vi "Programming Example Terahertz StepScan and FastScan.vi"() -> ()   [LabVIEW 2013]
uses:
  SubVIs/DeCoF SubVI Library/subVIs/DeCoF connection.ctl
  SubVIs/Commands.ctl
  SubVIs/Measurement.ctl
  SubVIs/Variables.ctl
  SubVIs/Store Data Actions.ctl
panel:
  in  "Set Bias to Zero":bool
  in  "Set Bias to Default":bool
  in  "IP Address of DLC smart":string="192.168.54.80"
  in  "Send All Values to DLC smart":bool
  out "Points Read":i32
  out "Fast-Scan-IsScanning":bool
  in  "FastScan":bool
  in  "Tx Amplitude":dbl caption="Tx Bias Amplitude (V)" step=0.1 format="%#.6g"
  in  "Tx Offset":dbl caption="Tx Bias Offset (V)" step=0.1 format="%#.6g"
  out "DLC smart Info":string
  in  "Int-Time(ms)":dbl=3.2768 caption="Integration Time (ms)" format="%#.6g"
  out "DLC smart Ok?":bool
  in  "Continuously":bool
  in  "Scan Selection":enum32{"No Selection", "Scan Up", "Scan Down"}(radio)
  in  "Quit App":bool
  in  "Max":dbl=650.0 caption="Max (GHz)"
  out "act.Step":dbl
  out "Graph Scan":T1(graph)
  in  "Step":dbl=0.002 caption="Step (GHz)" min=0.0 step=1e-05 format="%#_6f"
  in  "Min":dbl=600.0 caption="Min (GHz)"
  in  "Save Graph":bool
  in  "Clear Graph":bool
  out "Graph Samp":dbl[](graph)
  out "THz Cur":dbl caption="THz Current (nA)"
  in  "Gain Transimp. Amp.":dbl(ring)=1000000.0 caption="Transimp. Amp. Gain" items=["10^3 V/A"=1000.0, "10^4 V/A"=10000.0, "3.3 10^4 V/A  (1)"=33000.0, "10^5 V/A  (2)"=100000.0, "3.3 10^5 V/A  (3)"=330000.0, "10^6 V/A  (4)"=1000000.0, "3.3 10^6 V/A  (5)"=3300000.0, "10^7 V/A  (6)"=10000000.0]
  out "Connected?":bool
  in  "Sampling":bool
  in  "Freq.":dbl=600.0 caption="Frequency (GHz)" format="%#.6g"
  out "Connection ID":T2
  in  "Connect to DLC smart":bool
  in  "Laser Emission OnOff":bool
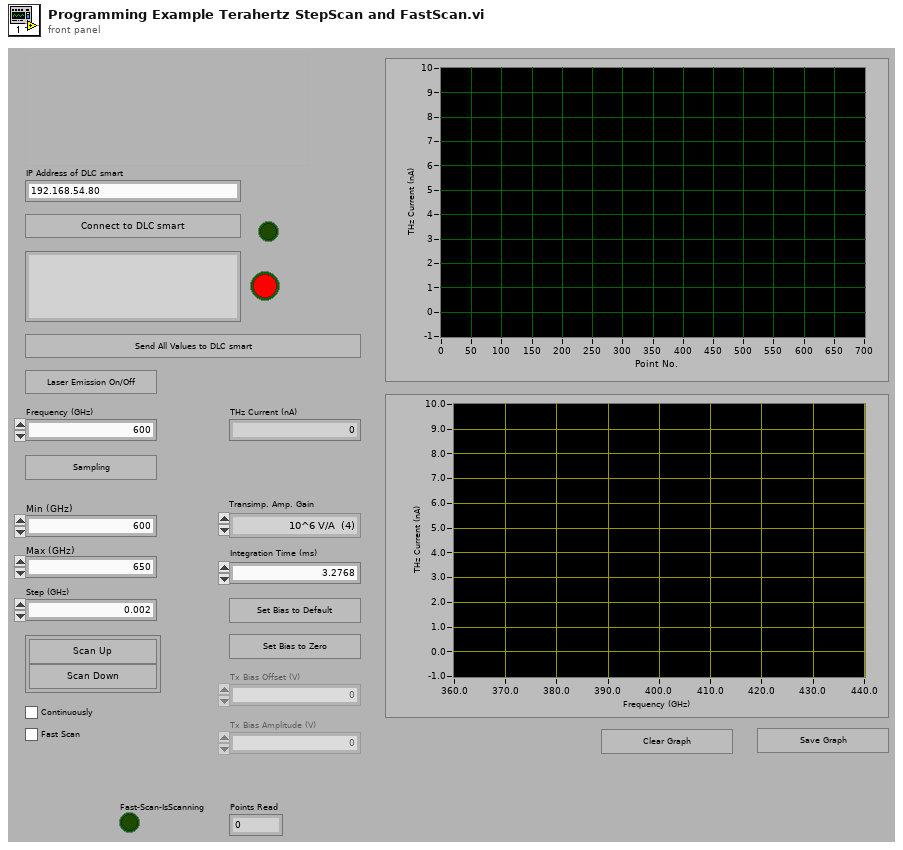
[diagram p1: front panel]
types:
  T1 = cluster{"array w/ subset deleted":dbl[], "array w/ subset deleted":dbl[]}
  T2 = typedef "DeCoF connection.ctl" = cluster{"TCP/IP":bool, "VISA":refnum<visa-resource-name>, "TCP/IP ID":refnum<k5>}
  T3 = typedef "Measurement.ctl" = enum16{"Init System", "Start Sampling", "Start Scan", "FastScan - Start", "FastScan - Get Data", "FastScan - Plot", "FastScan - End of Loop", "Precise - Set Frequency", "Precise - Reset Lock-In", "Precise - Wait", "Precise - Read Lock-In", "Precise - Store Data", "Precise - Plot", "Precise - End of Loop", "Stop Loop"}
  T4 = typedef "Commands.ctl" = enum16{"Init System", "Connect to DLC smart", "Verify DLC smart", "Laser Emission", "Send All Values to DLC smart", "Set Frequency", "Set FrequencyMin", "Set FrequencyMax", "Set FrequencyStep", "Set ScanModeFast", "Integration Time", "Set Bias to Default", "Set Bias to Zero", "Tx Bias Voltage", "Clear Graph", "Save Graph", "Clean Up"}
  T5 = typedef "Store Data Actions.ctl" = enum16{"Init", "Set", "Add", "Add Array", "Read", "Row+N"}
  T6 = typedef "Variables.ctl" = i32
  T7 = enum32{"invalid app kind", "Development System", "Run Time System", "Student Edition", "Embedded LabVIEW", "Evaluation", "Custom"}
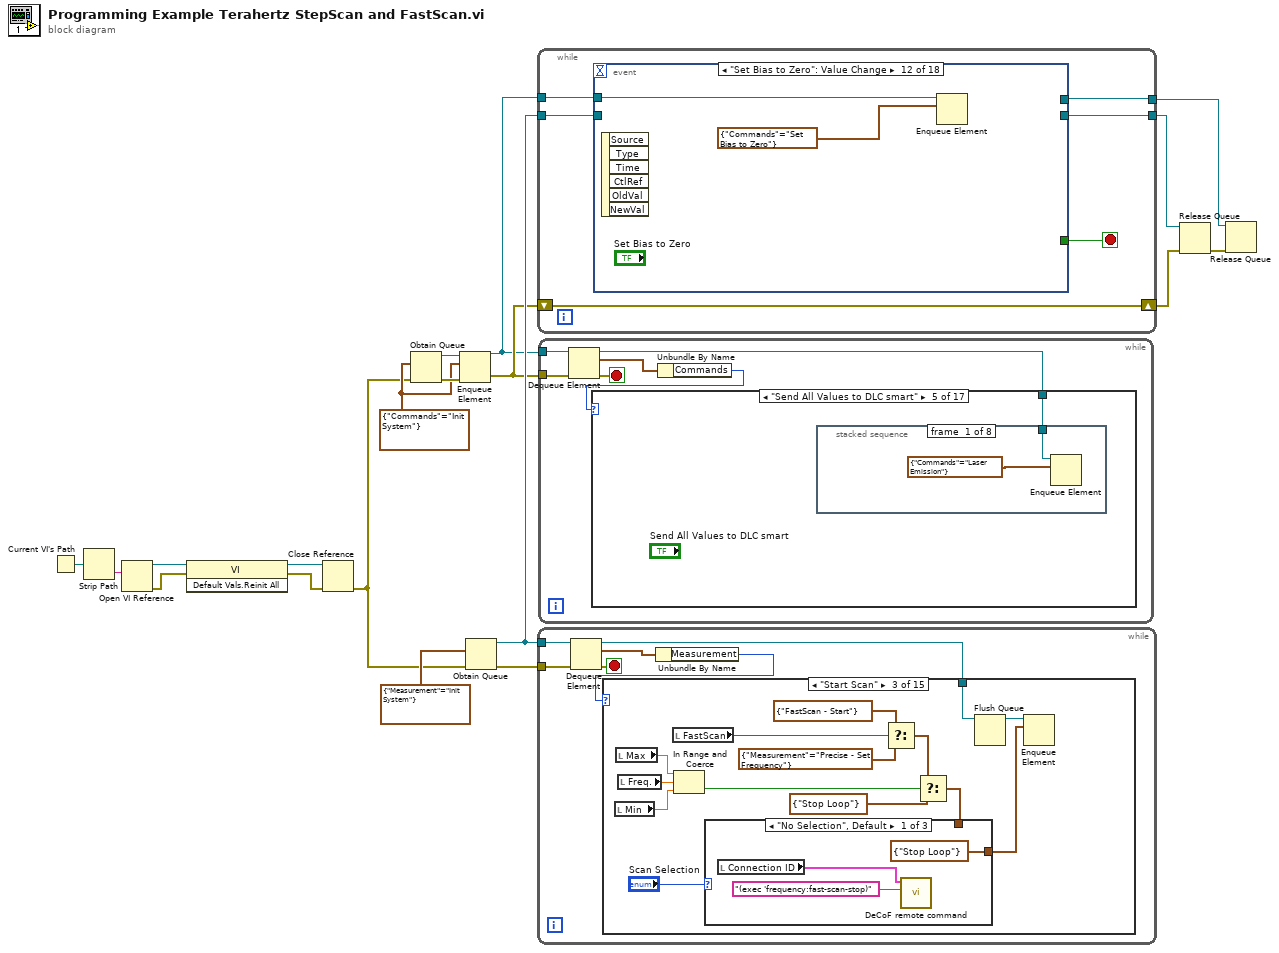
[diagram p0: block diagram]
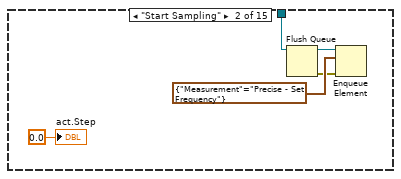
[diagram p3: hidden frame]
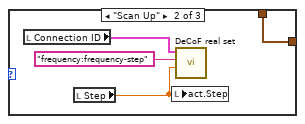
[diagram p4: hidden frame]
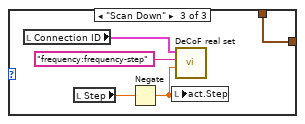
[diagram p5: hidden frame]
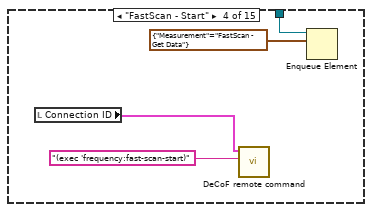
[diagram p6: hidden frame]
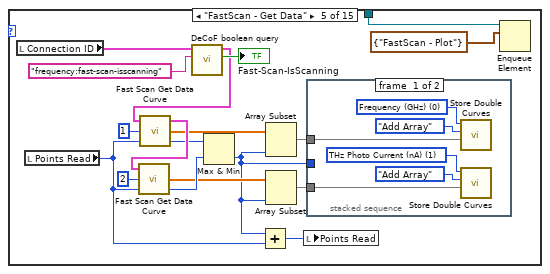
[diagram p7: hidden frame]
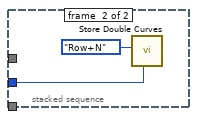
[diagram p8: hidden frame]
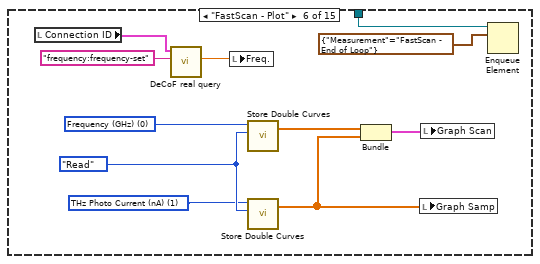
[diagram p9: hidden frame]
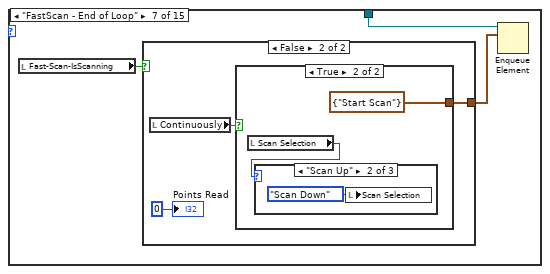
[diagram p10: hidden frame]
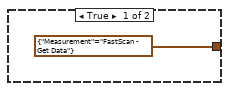
[diagram p11: hidden frame]
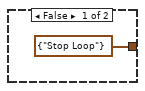
[diagram p12: hidden frame]
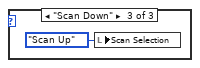
[diagram p14: hidden frame]
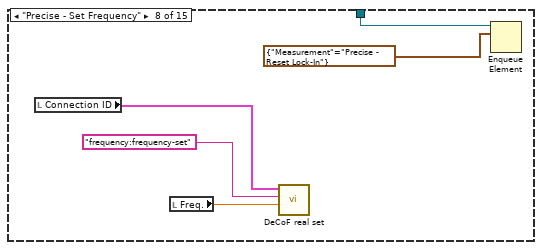
[diagram p15: hidden frame]
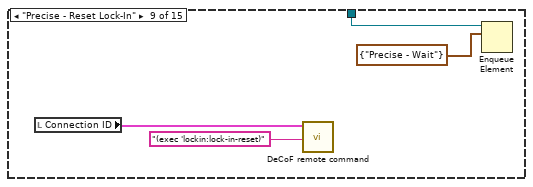
[diagram p16: hidden frame]
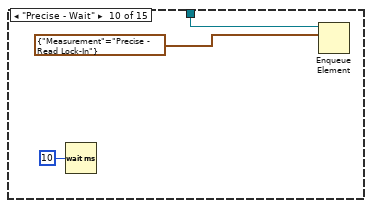
[diagram p17: hidden frame]
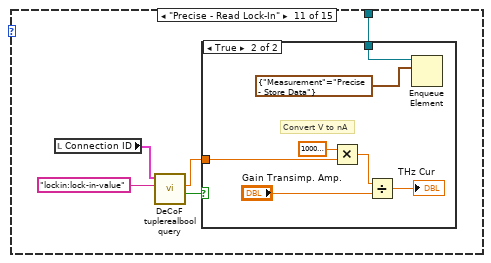
[diagram p18: hidden frame]
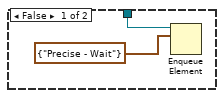
[diagram p19: hidden frame]
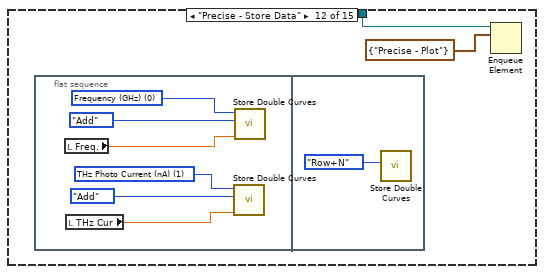
[diagram p20: hidden frame]
diagram:
  w16 = cluster{"Commands":T4} {"Commands"=enum."Init System"}
  n1 = Current VI's Path() -> (path=w10:path)
  n2 = Strip Path(path=w10) -> (name=w11:string)  [unwired: 1 out]
  n3 = Open VI Reference(vi path=w11) -> (vi reference=w9:refnum<vi>, error out=w13:errorcluster)  [unwired: 5 in]
  n4 = invoke class="VI" method="Default Vals.Reinit All"(reference=w9, error in=w13) -> (reference out=w12:refnum<vi>, error out=w14:errorcluster)  [unwired: 1 in, 1 out]
  n5 = Close Reference(reference=w12, error in (no error)=w14) -> (error out=w8:errorcluster)
  n6 = Obtain Queue(element data type=w16, error in (no error)=w8) -> (queue out=w19:refnum<queue>, error out=w18:errorcluster)  [unwired: 3 in, 1 out]
  n7 = Enqueue Element(queue=w19, element=w16, error in (no error)=w18) -> (queue out=w1:refnum<queue>, error out=w6:errorcluster)  [unwired: 1 in, 1 out]
  n8 = Obtain Queue(element data type=cluster{"Measurement":T3} {"Measurement"=enum."Init System"}, error in (no error)=w8) -> (queue out=w7:refnum<queue>, error out=w17:errorcluster)  [unwired: 3 in, 1 out]
  n9 = while {
    tunnel: w7 -> [w25]
    shift-right: [w21] -> w2
    shift-left: w6 -> [w21]
    tunnel: [w23] -> w4
    tunnel: [w22] -> w3
    tunnel: w1 -> [w20]
    stop <- w24 stop-if-true
    n10 = event shown="[11] \"Set Bias to Zero\": Value Change" {
      selector: _ -> [_ _ _ _ _ _ _ _ _ _ _ _ _ _ _ _ _ _]
      dyn-events: _ -> [_ _ _ _ _ _ _ _ _ _ _ _ _ _ _ _ _ _]
      timeout: _ -> [_ _ _ _ _ _ _ _ _ _ _ _ _ _ _ _ _ _]
      tunnel: w25 -> [_ _ _ _ _ _ _ _ _ _ _ _ _ w57 w60 _ _ w67]
      tunnel: [_ _ _ _ _ _ _ _ _ _ _ _ _ _ _ _ _ "Quit App"] -> w24
      tunnel: [_ _ _ _ _ _ _ _ _ _ _ _ _ _ _ _ _ w67] -> w23
      tunnel: [_ _ _ _ _ _ _ _ _ _ _ _ _ _ _ _ _ w66] -> w22
      tunnel: w20 -> [w26 w28 w30 w32 w34 w36 w38 w40 w42 w44 w46 w48 w50 _ _ w61 w63 w66]
      event "Connect to DLC smart": Value Change {
        n11 = event-data() -> ()  [unwired: 1 in, 5 out]
        n12 = Enqueue Element(queue=w26, element=cluster{"Commands":T4} {"Commands"=enum."Connect to DLC smart"}) -> ()  [unwired: 2 in, 3 out]
      }
      event "Save Graph": Value Change {
        n13 = event-data() -> ()  [unwired: 1 in, 5 out]
        n14 = Enqueue Element(queue=w28, element=cluster{"Commands":T4} {"Commands"=enum."Save Graph"}) -> ()  [unwired: 2 in, 3 out]
      }
      event "Laser Emission OnOff": Value Change {
        n15 = event-data() -> ()  [unwired: 1 in, 6 out]
        n16 = Enqueue Element(queue=w30, element=cluster{"Commands":T4} {"Commands"=enum."Laser Emission"}) -> ()  [unwired: 2 in, 3 out]
      }
      event "Send All Values to DLC smart": Value Change {
        n17 = event-data() -> ()  [unwired: 1 in, 6 out]
        n18 = Enqueue Element(queue=w32, element=cluster{"Commands":T4} {"Commands"=enum."Send All Values to DLC smart"}) -> ()  [unwired: 2 in, 3 out]
      }
      event "Freq.": Value Change {
        n19 = event-data() -> ()  [unwired: 1 in, 6 out]
        n20 = Enqueue Element(queue=w34, element=cluster{"Commands":T4} {"Commands"=enum."Set Frequency"}) -> ()  [unwired: 2 in, 3 out]
      }
      event "Min": Value Change {
        n21 = event-data() -> ()  [unwired: 1 in, 6 out]
        n22 = Enqueue Element(queue=w36, element=cluster{"Commands":T4} {"Commands"=enum."Set FrequencyMin"}) -> ()  [unwired: 2 in, 3 out]
      }
      event "Max": Value Change {
        n23 = event-data() -> ()  [unwired: 1 in, 6 out]
        n24 = Enqueue Element(queue=w38, element=cluster{"Commands":T4} {"Commands"=enum."Set FrequencyMax"}) -> ()  [unwired: 2 in, 3 out]
      }
      event "Step": Value Change {
        n25 = event-data() -> ()  [unwired: 1 in, 6 out]
        n26 = Enqueue Element(queue=w40, element=cluster{"Commands":T4} {"Commands"=enum."Set FrequencyStep"}) -> ()  [unwired: 2 in, 3 out]
      }
      event "FastScan": Value Change {
        n27 = event-data() -> ()  [unwired: 1 in, 6 out]
        n28 = Enqueue Element(queue=w42, element=cluster{"Commands":T4} {"Commands"=enum."Set ScanModeFast"}) -> ()  [unwired: 2 in, 3 out]
      }
      event "Int-Time(ms)": Value Change {
        n29 = event-data() -> ()  [unwired: 1 in, 6 out]
        n30 = Enqueue Element(queue=w44, element=cluster{"Commands":T4} {"Commands"=enum."Integration Time"}) -> ()  [unwired: 2 in, 3 out]
      }
      event "Set Bias to Default": Value Change {
        n31 = event-data() -> ()  [unwired: 1 in, 6 out]
        n32 = Enqueue Element(queue=w46, element=cluster{"Commands":T4} {"Commands"=enum."Set Bias to Default"}) -> ()  [unwired: 2 in, 3 out]
      }
      event "Set Bias to Zero": Value Change {
        n33 = event-data() -> ()  [unwired: 1 in, 6 out]
        n34 = Enqueue Element(queue=w48, element=cluster{"Commands":T4} {"Commands"=enum."Set Bias to Zero"}) -> ()  [unwired: 2 in, 3 out]
      }
      event "Tx Offset", "Tx Amplitude": Value Change {
        n35 = event-data() -> ()  [unwired: 1 in, 6 out]
        n36 = Enqueue Element(queue=w50, element=cluster{"Commands":T4} {"Commands"=enum."Tx Bias Voltage"}) -> ()  [unwired: 2 in, 3 out]
      }
      event "Sampling": Value Change {
        n37 = event-data() -> ("NewVal"=w56:bool)  [unwired: 1 in, 5 out]
        n38 = local write "Scan Selection"(enum32{"No Selection", "Scan Up", "Scan Down"}."No Selection" ("Scan Selection")) -> ()
        n39 = Select(t=cluster{"Measurement":T3} {"Measurement"=enum."Start Sampling"}, s=w56, f=cluster{"Measurement":T3} {"Measurement"=enum."Stop Loop"} ("element")) -> (s? t:f=w54:cluster{"Measurement":T3})
        n40 = Enqueue Element(queue=w57, element=w54) -> ()  [unwired: 2 in, 3 out]
      }
      event "Scan Selection": Value Change {
        n41 = event-data() -> ()  [unwired: 1 in, 6 out]
        n42 = local write "Sampling"(FALSE ("Start Scan UI")) -> ()
        n43 = Enqueue Element(queue=w60, element=cluster{"Measurement":T3} {"Measurement"=enum."Start Scan"}) -> ()  [unwired: 2 in, 3 out]
      }
      event "Clear Graph": Value Change {
        n44 = event-data() -> ()  [unwired: 1 in, 5 out]
        n45 = Enqueue Element(queue=w61, element=cluster{"Commands":T4} {"Commands"=enum."Clear Graph"}) -> ()  [unwired: 2 in, 3 out]
      }
      event Panel Close? {
        n46 = event-data() -> ()  [unwired: 1 in, 3 out]
        n47 = Enqueue Element(queue=w63, element=cluster{"Commands":T4} {"Commands"=enum."Clean Up"}) -> ()  [unwired: 2 in, 3 out]
        n48 = event-data("Discard?"=TRUE ("stop")) -> ()  [unwired: 1 in, 1 out]
      }
      event "Quit App": Value Change {
        n49 = event-data() -> ()  [unwired: 1 in, 5 out]
      }
    }
  }
  n50 = while {
    tunnel: w7 -> [w74]
    tunnel: w17 -> [w73]
    stop <- w72 stop-if-true
    n51 = Dequeue Element(queue=w74, error in (no error)=w73) -> (queue out=w70:refnum<queue>, element=w69:cluster{"Measurement":T3}, error out=w72:errorcluster)  [unwired: 1 in, 1 out]
    n52 = Unbundle By Name(w69) -> ("Measurement"=w71:T3)
    n53 = case shown="\"Start Scan\"" w71 {
      tunnel: w70 -> [_ w78 w93 w109 w127 w146 w149 w162 w165 w169 w175 w186 w201 w211 w224]
      frame "Init System" {
      }
      frame "Start Sampling" {
        n54 = Flush Queue(queue=w78) -> (queue out=w77:refnum<queue>, error out=w76:errorcluster)  [unwired: 1 in, 1 out]
        n55 = Enqueue Element(queue=w77, element=cluster{"Measurement":T3} {"Measurement"=enum."Precise - Set Frequency"}, error in (no error)=w76) -> ()  [unwired: 1 in, 3 out]
        "act.Step" <- 0.0 ("act.Step")
      }
      frame "Start Scan" {
        n56 = local read "Min"() -> (w89:dbl)
        n57 = local read "Max"() -> (w90:dbl)
        n58 = local read "Freq."() -> (w91:dbl)
        n59 = local read "FastScan"() -> (w83:bool)
        n60 = In Range and Coerce(upper limit=w90, x=w91, lower limit=w89) -> (In Range?=w87:bool)  [unwired: 1 out]
        n61 = Select(t=cluster{"Measurement":T3} {"Measurement"=enum."FastScan - Start"}, s=w83, f=cluster{"Measurement":T3} {"Measurement"=enum."Precise - Set Frequency"} ("element")) -> (s? t:f=w86:cluster{"Measurement":T3})
        n62 = Select(t=w86, s=w87, f=cluster{"Measurement":T3} {"Measurement"=enum."Stop Loop"} ("element")) -> (s? t:f=w82:cluster{"Measurement":T3})
        n63 = case shown="\"No Selection\", Default" "Scan Selection" {
          tunnel: w82 -> [_ w100 w104]
          tunnel: [cluster{"Measurement":T3} {"Measurement"=enum."Stop Loop"} ("element") w100 w104] -> w81
          frame "No Selection", Default {
            n64 = local read "Connection ID"() -> (w94:T2)
            n65 = call "DeCoF remote command.vi"("command"="(exec 'frequency:fast-scan-stop)" ("param-name"), "Conncection ID in"=w94) -> ()  [unwired: 3 in, 5 out]
          }
          frame "Scan Up" {
            n66 = local read "Connection ID"() -> (w98:T2)
            n67 = local read "Step"() -> (w97:dbl)
            n68 = local write "act.Step"(w97) -> ()
            n69 = call "DeCoF real set.vi"("value"=w97, "param-name"="frequency:frequency-step", "Conncection ID in"=w98) -> ()  [unwired: 3 in, 2 out]
          }
          frame "Scan Down" {
            n70 = local read "Connection ID"() -> (w102:T2)
            n71 = local read "Step"() -> (w105:dbl)
            n72 = Negate(x=w105) -> (-x=w101:dbl)
            n73 = local write "act.Step"(w101) -> ()
            n74 = call "DeCoF real set.vi"("value"=w101, "param-name"="frequency:frequency-step", "Conncection ID in"=w102) -> ()  [unwired: 3 in, 2 out]
          }
        }
        n75 = Flush Queue(queue=w93) -> (queue out=w92:refnum<queue>)  [unwired: 1 in, 2 out]
        n76 = Enqueue Element(queue=w92, element=w81) -> ()  [unwired: 2 in, 3 out]
      }
      frame "FastScan - Start" {
        n77 = local read "Connection ID"() -> (w106:T2)
        n78 = call "DeCoF remote command.vi"("command"="(exec 'frequency:fast-scan-start)" ("param-name"), "Conncection ID in"=w106) -> ()  [unwired: 3 in, 5 out]
        n79 = Enqueue Element(queue=w109, element=cluster{"Measurement":T3} {"Measurement"=enum."FastScan - Get Data"}) -> ()  [unwired: 2 in, 3 out]
      }
      frame "FastScan - Get Data" {
        n80 = local read "Connection ID"() -> (w126:T2)
        n81 = local read "Points Read"() -> (w112:i32)
        n82 = call "DeCoF boolean query.vi"("param-name"="frequency:fast-scan-isscanning", "Conncection ID in"=w126) -> ("value"=→"Fast-Scan-IsScanning":bool, "Conncection ID out"=w122:T2)  [unwired: 3 in, 1 out]
        n83 = call "Fast Scan Get Data Curve.vi"("Start Index"=w112, "Curve Number"=1, "Conncection ID in"=w122) -> ("Size of Double Array"=w118:i32, "Double Array"=w116:dbl[], "Conncection ID out"=w120:T2)
        n84 = call "Fast Scan Get Data Curve.vi"("Start Index"=w112, "Curve Number"=2, "Conncection ID in"=w120) -> ("Size of Double Array"=w117:i32, "Double Array"=w115:dbl[])  [unwired: 1 out]
        n85 = Max & Min(x=w118, y=w117) -> (min(x,y)=w110:i32)  [unwired: 1 out]
        n86 = Add(x=w110, y=w112) -> (x+y=w111:i32)
        n87 = Array Subset(array=w116, length=w110) -> (w114:dbl[])  [unwired: 1 in]
        n88 = Array Subset(array=w115, length=w110) -> (w113:dbl[])  [unwired: 1 in]
        n89 = local write "Points Read"(w111) -> ()
        n90 = stacked-sequence {
          tunnel: w114 -> [w133 _]
          tunnel: w113 -> [w128 _]
          tunnel: w110 -> [_ w134]
          frame #0 {
            w130 = T6 1 items=["Frequency (GHz)", "THz Photo Current (nA)"] ("Curve Index")
            w131 = T6 0 items=["Frequency (GHz)", "THz Photo Current (nA)"] ("Curve Index")
            n91 = call "Store Double Curves.vi"("Array in"=w133, "Action"=Store_Data_Actions."Add Array", "Curve Index"=w131) -> ()  [unwired: 3 in, 2 out]
            n92 = call "Store Double Curves.vi"("Array in"=w128, "Action"=Store_Data_Actions."Add Array", "Curve Index"=w130) -> ()  [unwired: 3 in, 2 out]
          }
          frame #1 {
            n93 = call "Store Double Curves.vi"("N"=w134, "Action"=Store_Data_Actions."Row+N") -> ()  [unwired: 4 in, 2 out]
          }
        }
        n94 = Enqueue Element(queue=w127, element=cluster{"Measurement":T3} {"Measurement"=enum."FastScan - Plot"}) -> ()  [unwired: 2 in, 3 out]
      }
      frame "FastScan - Plot" {
        w142 = T6 0 items=["Frequency (GHz)", "THz Photo Current (nA)"] ("Curve Index")
        w143 = T6 1 items=["Frequency (GHz)", "THz Photo Current (nA)"] ("Curve Index")
        w144 = Store_Data_Actions."Read" ("Action")
        n95 = local read "Connection ID"() -> (w138:T2)
        n96 = call "DeCoF real query.vi"("param-name"="frequency:frequency-set", "Conncection ID in"=w138) -> ("value"=w136:dbl)  [unwired: 3 in, 2 out]
        n97 = local write "Freq."(w136) -> ()
        n98 = call "Store Double Curves.vi"("Action"=w144, "Curve Index"=w142) -> ("Array out"=w141:dbl[])  [unwired: 4 in, 1 out]
        n99 = call "Store Double Curves.vi"("Action"=w144, "Curve Index"=w143) -> ("Array out"=w139:dbl[])  [unwired: 4 in, 1 out]
        n100 = Bundle("Array out"=w141, "Array out"=w139) -> (w140:cluster{"Array out":dbl[], "Array out":dbl[]})  [unwired: 1 in]
        n101 = local write "Graph Samp"(w139) -> ()
        n102 = local write "Graph Scan"(w140) -> ()
        n103 = Enqueue Element(queue=w146, element=cluster{"Measurement":T3} {"Measurement"=enum."FastScan - End of Loop"}) -> ()  [unwired: 2 in, 3 out]
      }
      frame "FastScan - End of Loop" {
        n104 = local read "Fast-Scan-IsScanning"() -> (w148:bool)
        n105 = case shown="False" w148 {
          tunnel: [cluster{"Measurement":T3} {"Measurement"=enum."FastScan - Get Data"} ("element") w152] -> w147
          frame True {
          }
          frame False {
            n106 = local read "Continuously"() -> (w153:bool)
            n107 = case shown="True" w153 {
              tunnel: [cluster{"Measurement":T3} {"Measurement"=enum."Stop Loop"} ("element") cluster{"Measurement":T3} {"Measurement"=enum."Start Scan"} ("element")] -> w152
              frame False {
              }
              frame True {
                n108 = local read "Scan Selection"() -> (w156:enum32{"No Selection", "Scan Up", "Scan Down"})
                n109 = case shown="\"Scan Up\"" w156 {
                  frame "No Selection", Default {
                  }
                  frame "Scan Up" {
                    n110 = local write "Scan Selection"(enum32{"No Selection", "Scan Up", "Scan Down"}."Scan Down" ("Scan Selection")) -> ()
                  }
                  frame "Scan Down" {
                    n111 = local write "Scan Selection"(enum32{"No Selection", "Scan Up", "Scan Down"}."Scan Up" ("Scan Selection")) -> ()
                  }
                }
              }
            }
            "Points Read" <- 0 ("Points Read")
          }
        }
        n112 = Enqueue Element(queue=w149, element=w147) -> ()  [unwired: 2 in, 3 out]
      }
      frame "Precise - Set Frequency" {
        n113 = local read "Connection ID"() -> (w160:T2)
        n114 = local read "Freq."() -> (w159:dbl)
        n115 = call "DeCoF real set.vi"("value"=w159, "param-name"="frequency:frequency-set", "Conncection ID in"=w160) -> ()  [unwired: 3 in, 2 out]
        n116 = Enqueue Element(queue=w162, element=cluster{"Measurement":T3} {"Measurement"=enum."Precise - Reset Lock-In"}) -> ()  [unwired: 2 in, 3 out]
      }
      frame "Precise - Reset Lock-In" {
        n117 = local read "Connection ID"() -> (w164:T2)
        n118 = call "DeCoF remote command.vi"("command"="(exec 'lockin:lock-in-reset)" ("format string"), "Conncection ID in"=w164) -> ()  [unwired: 3 in, 5 out]
        n119 = Enqueue Element(queue=w165, element=cluster{"Measurement":T3} {"Measurement"=enum."Precise - Wait"}) -> ()  [unwired: 2 in, 3 out]
      }
      frame "Precise - Wait" {
        n120 = Wait (ms)(milliseconds to wait=u32 10) -> ()  [unwired: 1 out]
        n121 = Enqueue Element(queue=w169, element=cluster{"Measurement":T3} {"Measurement"=enum."Precise - Read Lock-In"}) -> ()  [unwired: 2 in, 3 out]
      }
      frame "Precise - Read Lock-In" {
        n122 = local read "Connection ID"() -> (w171:T2)
        n123 = call "DeCoF tuplerealbool query.vi"("param-name"="lockin:lock-in-value" ("format string"), "Conncection ID in"=w171) -> ("boolean value"=w173:bool, "real value"=w174:dbl)  [unwired: 2 in, 2 out]
        n124 = case shown="True" w173 {
          tunnel: w175 -> [w177 w180]
          tunnel: w174 -> [_ w184]
          frame False {
            n125 = Enqueue Element(queue=w177, element=cluster{"Measurement":T3} {"Measurement"=enum."Precise - Wait"}) -> ()  [unwired: 2 in, 3 out]
          }
          frame True {
            # "Convert V to nA"
            n126 = Multiply(x=1000000000.0 ("y"), y=w184) -> (x*y=w183:dbl)
            n127 = Divide(x=w183, y="Gain Transimp. Amp.") -> (x/y=→"THz Cur":dbl)
            n128 = Enqueue Element(queue=w180, element=cluster{"Measurement":T3} {"Measurement"=enum."Precise - Store Data"}) -> ()  [unwired: 2 in, 3 out]
          }
        }
      }
      frame "Precise - Store Data" {
        n129 = flat-sequence {
          frame #0 {
            w188 = T6 0 items=["Frequency (GHz)", "THz Photo Current (nA)"] ("Curve Index")
            w187 = T6 1 items=["Frequency (GHz)", "THz Photo Current (nA)"] ("Curve Index")
            n130 = local read "Freq."() -> (w190:dbl)
            n131 = local read "THz Cur"() -> (w189:dbl)
            n132 = call "Store Double Curves.vi"("Element in"=w189, "Action"=Store_Data_Actions."Add", "Curve Index"=w187) -> ()  [unwired: 3 in, 2 out]
            n133 = call "Store Double Curves.vi"("Element in"=w190, "Action"=Store_Data_Actions."Add", "Curve Index"=w188) -> ()  [unwired: 3 in, 2 out]
          }
          frame #1 {
            n134 = call "Store Double Curves.vi"("Action"=Store_Data_Actions."Row+N") -> ()  [unwired: 5 in, 2 out]
          }
        }
        n135 = Enqueue Element(queue=w186, element=cluster{"Measurement":T3} {"Measurement"=enum."Precise - Plot"}) -> ()  [unwired: 2 in, 3 out]
      }
      frame "Precise - Plot" {
        w196 = T6 0 items=["Frequency (GHz)", "THz Photo Current (nA)"] ("Curve Index")
        w198 = T6 1 items=["Frequency (GHz)", "THz Photo Current (nA)"] ("Curve Index")
        w199 = Store_Data_Actions."Read" ("Action")
        n136 = call "Store Double Curves.vi"("Action"=w199, "Curve Index"=w196) -> ("Array out"=w195:dbl[])  [unwired: 4 in, 1 out]
        n137 = call "Store Double Curves.vi"("Action"=w199, "Curve Index"=w198) -> ("Array out"=w194:dbl[])  [unwired: 4 in, 1 out]
        "Graph Samp" <- w194
        n138 = Bundle("Array out"=w195, "Array out"=w194) -> (→"Graph Scan":cluster{"Array out":dbl[], "Array out":dbl[]})  [unwired: 1 in]
        n139 = Enqueue Element(queue=w201, element=cluster{"Measurement":T3} {"Measurement"=enum."Precise - End of Loop"}) -> ()  [unwired: 2 in, 3 out]
      }
      frame "Precise - End of Loop" {
        n140 = local read "Min"() -> (w206:dbl)
        n141 = local read "Max"() -> (w207:dbl)
        n142 = local read "Freq."() -> (w209:dbl)
        n143 = local read "act.Step"() -> (w210:dbl)
        n144 = Add(x=w209, y=w210) -> (x+y=w202:dbl)
        n145 = In Range and Coerce(upper limit=w207, x=w202, lower limit=w206) -> (In Range?=w205:bool)  [unwired: 1 out]
        n146 = Or(x="Sampling", y=w205) -> (x .or. y?=w204:bool)
        n147 = case shown="False" w204 {
          tunnel: [w212 cluster{"Measurement":T3} {"Measurement"=enum."Precise - Set Frequency"} ("t")] -> w203
          tunnel: w202 -> [_ w219]
          frame False {
            n148 = case shown="True" "Continuously" {
              tunnel: [cluster{"Measurement":T3} {"Measurement"=enum."Stop Loop"} ("f") cluster{"Measurement":T3} {"Measurement"=enum."Start Scan"} ("element")] -> w212
              frame False {
              }
              frame True {
                n149 = local read "Scan Selection"() -> (w215:enum32{"No Selection", "Scan Up", "Scan Down"})
                n150 = case shown="\"Scan Up\"" w215 {
                  frame "No Selection", Default {
                  }
                  frame "Scan Up" {
                    n151 = local write "Scan Selection"(enum32{"No Selection", "Scan Up", "Scan Down"}."Scan Down" ("Scan Selection")) -> ()
                  }
                  frame "Scan Down" {
                    n152 = local write "Scan Selection"(enum32{"No Selection", "Scan Up", "Scan Down"}."Scan Up" ("Scan Selection")) -> ()
                  }
                }
              }
            }
          }
          frame True {
            n153 = local write "Freq."(w219) -> ()
          }
        }
        n154 = Enqueue Element(queue=w211, element=w203) -> ()  [unwired: 2 in, 3 out]
      }
      frame "Stop Loop" {
        n155 = local write "Scan Selection"(enum32{"No Selection", "Scan Up", "Scan Down"}."No Selection" ("Scan Selection")) -> ()
        n156 = local write "Points Read"(0 ("Points Read")) -> ()
        n157 = local write "Sampling"(FALSE ("Start Scan")) -> ()
        n158 = Flush Queue(queue=w224) -> ()  [unwired: 1 in, 3 out]
      }
    }
  }
  n159 = while {
    tunnel: w1 -> [w230]
    tunnel: w6 -> [w228]
    stop <- w229 stop-if-true
    n160 = Dequeue Element(queue=w230, error in (no error)=w228) -> (queue out=w227:refnum<queue>, element=w226:cluster{"Commands":T4}, error out=w229:errorcluster)  [unwired: 1 in, 1 out]
    n161 = Unbundle By Name(w226) -> ("Commands"=w225:T4)
    n162 = case shown="\"Send All Values to DLC smart\"" w225 {
      tunnel: w227 -> [_ w241 _ _ w262 _ _ _ _ _ _ _ _ _ _ _ _]
      frame "Init System", Default {
        n163 = call "Store Double Curves.vi"("Action"=Store_Data_Actions."Init") -> ()  [unwired: 5 in, 2 out]
      }
      frame "Connect to DLC smart" {
        n164 = Concatenate Strings("IP Address of DLC smart", ":1998" ("address")) -> (w232:string)
        n165 = call "DeCoF open connection.vi"("TCP?"=TRUE, "address"=w232) -> ("error out"=w237:errorcluster, "Conncection ID out"=→"Connection ID":T2)  [unwired: 4 in]
        n166 = Unbundle By Name(w237) -> ("status"=w240:bool)
        n167 = Not(x=w240) -> (.not. x?=→"Connected?":bool)
        n168 = Enqueue Element(queue=w241, element=cluster{"Commands":T4} {"Commands"=enum."Verify DLC smart"}) -> ()  [unwired: 2 in, 3 out]
      }
      frame "Verify DLC smart" {
        w243 = "\r\n"
        w244 = ")" ("string")
        w246 = "(Expected: " ("string")
        w245 = "2.2.1.8799"
        w249 = "DLCsmartTHz"
        n169 = local read "Connection ID"() -> (w258:T2)
        n170 = call "DeCoF string query.vi"("param-name"="general:system-type", "Conncection ID in"=w258) -> ("value"=w255:string, "Conncection ID out"=w256:T2)  [unwired: 3 in, 1 out]
        n171 = Equal?(x=w255, y=w249) -> (x = y?=w253:bool)
        n172 = call "DeCoF string query.vi"("param-name"="general:fw-ver", "Conncection ID in"=w256) -> ("value"=w247:string)  [unwired: 3 in, 2 out]
        n173 = Equal?(x=w247, y=w245) -> (x = y?=w252:bool)
        n174 = And(x=w253, y=w252) -> (x .and. y?=→"DLC smart Ok?":bool)
        n175 = Concatenate Strings("general:system-type: ", w255, w243, w246, w249, w244, w243, "general:fw-ver: " ("string"), w247, w243, w246, w245, w244) -> (→"DLC smart Info":string)
      }
      frame "Laser Emission" {
        n176 = local read "Connection ID"() -> (w259:T2)
        n177 = call "DeCoF boolean set.vi"("value"="Laser Emission OnOff", "param-name"="laser-operation:emission-global-enable", "Conncection ID in"=w259) -> ()  [unwired: 3 in, 2 out]
      }
      frame "Send All Values to DLC smart" {
        n178 = stacked-sequence {
          tunnel: w262 -> [w263 w265 w267 w269 w271 w273 w275 w277]
          frame #0 {
            n179 = Enqueue Element(queue=w263, element=cluster{"Commands":T4} {"Commands"=enum."Laser Emission"}) -> ()  [unwired: 2 in, 3 out]
          }
          frame #1 {
            n180 = Enqueue Element(queue=w265, element=cluster{"Commands":T4} {"Commands"=enum."Set Frequency"}) -> ()  [unwired: 2 in, 3 out]
          }
          frame #2 {
            n181 = Enqueue Element(queue=w267, element=cluster{"Commands":T4} {"Commands"=enum."Set FrequencyMin"}) -> ()  [unwired: 2 in, 3 out]
          }
          frame #3 {
            n182 = Enqueue Element(queue=w269, element=cluster{"Commands":T4} {"Commands"=enum."Set FrequencyMax"}) -> ()  [unwired: 2 in, 3 out]
          }
          frame #4 {
            n183 = Enqueue Element(queue=w271, element=cluster{"Commands":T4} {"Commands"=enum."Set FrequencyStep"}) -> ()  [unwired: 2 in, 3 out]
          }
          frame #5 {
            n184 = Enqueue Element(queue=w273, element=cluster{"Commands":T4} {"Commands"=enum."Set ScanModeFast"}) -> ()  [unwired: 2 in, 3 out]
          }
          frame #6 {
            n185 = Enqueue Element(queue=w275, element=cluster{"Commands":T4} {"Commands"=enum."Integration Time"}) -> ()  [unwired: 2 in, 3 out]
          }
          frame #7 {
            n186 = Enqueue Element(queue=w277, element=cluster{"Commands":T4} {"Commands"=enum."Tx Bias Voltage"}) -> ()  [unwired: 2 in, 3 out]
          }
        }
      }
      frame "Set Frequency" {
        n187 = local read "Connection ID"() -> (w280:T2)
        n188 = call "DeCoF real set.vi"("value"="Freq.", "param-name"="frequency:frequency-set", "Conncection ID in"=w280) -> ()  [unwired: 3 in, 2 out]
      }
      frame "Set FrequencyMin" {
        n189 = local read "Connection ID"() -> (w284:T2)
        n190 = call "DeCoF real set.vi"("value"="Min", "param-name"="frequency:frequency-min", "Conncection ID in"=w284) -> ()  [unwired: 3 in, 2 out]
      }
      frame "Set FrequencyMax" {
        n191 = local read "Connection ID"() -> (w287:T2)
        n192 = call "DeCoF real set.vi"("value"="Max", "param-name"="frequency:frequency-max", "Conncection ID in"=w287) -> ()  [unwired: 3 in, 2 out]
      }
      frame "Set FrequencyStep" {
      }
      frame "Set ScanModeFast" {
        n193 = local read "Connection ID"() -> (w289:T2)
        n194 = call "DeCoF boolean set.vi"("value"="FastScan", "param-name"="frequency:scan-mode-fast", "Conncection ID in"=w289) -> ()  [unwired: 3 in, 2 out]
      }
      frame "Integration Time" {
        w292 = "lockin:integration-time" ("param-name")
        n195 = local read "Connection ID"() -> (w295:T2)
        n196 = call "DeCoF real set.vi"("value"="Int-Time(ms)", "param-name"=w292, "Conncection ID in"=w295) -> ("Conncection ID out"=w293:T2)  [unwired: 3 in, 1 out]
        n197 = call "DeCoF real query.vi"("param-name"=w292, "Conncection ID in"=w293) -> ("value"=w291:dbl)  [unwired: 3 in, 2 out]
        n198 = local write "Int-Time(ms)"(w291) -> ()
      }
      frame "Set Bias to Default" {
        n199 = local read "Connection ID"() -> (w303:T2)
        n200 = call "DeCoF remote command.vi"("command"="(exec 'lockin:mod-out-set-to-default)" ("param-name"), "Conncection ID in"=w303) -> ("Conncection ID out"=w301:T2)  [unwired: 3 in, 4 out]
        n201 = call "DeCoF real query.vi"("param-name"="lockin:mod-out-offset", "Conncection ID in"=w301) -> ("value"=w297:dbl, "Conncection ID out"=w299:T2)  [unwired: 3 in, 1 out]
        n202 = local write "Tx Offset"(w297) -> ()
        n203 = call "DeCoF real query.vi"("param-name"="lockin:mod-out-amplitude", "Conncection ID in"=w299) -> ("value"=w296:dbl)  [unwired: 3 in, 2 out]
        n204 = local write "Tx Amplitude"(w296) -> ()
      }
      frame "Set Bias to Zero" {
        n205 = local read "Connection ID"() -> (w311:T2)
        n206 = call "DeCoF remote command.vi"("command"="(exec 'lockin:mod-out-set-to-zero)" ("param-name"), "Conncection ID in"=w311) -> ("Conncection ID out"=w309:T2)  [unwired: 3 in, 4 out]
        n207 = call "DeCoF real query.vi"("param-name"="lockin:mod-out-offset", "Conncection ID in"=w309) -> ("value"=w305:dbl, "Conncection ID out"=w307:T2)  [unwired: 3 in, 1 out]
        n208 = local write "Tx Offset"(w305) -> ()
        n209 = call "DeCoF real query.vi"("param-name"="lockin_mod-out-amplitude", "Conncection ID in"=w307) -> ("value"=w304:dbl)  [unwired: 3 in, 2 out]
        n210 = local write "Tx Amplitude"(w304) -> ()
      }
      frame "Tx Bias Voltage" {
        n211 = local read "Connection ID"() -> (w317:T2)
        n212 = call "DeCoF real set.vi"("value"="Tx Offset", "param-name"="lockin:mod-out-offset ", "Conncection ID in"=w317) -> ("Conncection ID out"=w316:T2)  [unwired: 3 in, 1 out]
        n213 = call "DeCoF real set.vi"("value"="Tx Amplitude", "param-name"="lockin:mod-out-amplitude ", "Conncection ID in"=w316) -> ()  [unwired: 3 in, 2 out]
      }
      frame "Clear Graph" {
        n214 = invoke on="Graph Samp" class="WaveformGraph (strict)" method="Reinit To Default"() -> ()  [unwired: 3 in, 3 out]
        n215 = call "Store Double Curves.vi"("Action"=Store_Data_Actions."Init") -> ()  [unwired: 5 in, 2 out]
        n216 = invoke on="Graph Scan" class="XYGraph (strict)" method="Reinit To Default"() -> ()  [unwired: 3 in, 3 out]
      }
      frame "Save Graph" {
        n217 = Concatenate Strings("Frequency (GHz)" ("string"), "\t", "THz Current (nA)" ("string"), "\r\n") -> (w319:string)
        n218 = call "Create Store Array.vi"() -> ("Array"=w320:dbl[][])  [unwired: 5 in]
        n219 = call "Write To Spreadsheet File_extended.vi"("transpose? (no:F)"=TRUE ("append to file? (new file:F)"), "header"=w319, "2D data"=w320) -> ()  [unwired: 7 in, 1 out]
      }
      frame "Clean Up" {
        n220 = local read "Connection ID"() -> (w332:T2)
        n221 = call "DeCoF close connection.vi"("Connection ID in"=w332) -> ("error out"=w329:errorcluster)  [unwired: 5 in, 1 out]
        n222 = property on="Quit App" class="Bool (strict)"(error in=w329, "Val(Sgnl)"=TRUE) -> (error out=w330:errorcluster)  [unwired: 1 in, 1 out]
        n223 = property class="App"(error in=w330) -> ("App.Kind"=w327:T7)  [unwired: 1 in, 2 out]
        n224 = Equal?(x=T7."Run Time System", y=w327) -> (x = y?=w331:bool)
        n225 = Quit LabVIEW(quit? (T)=w331) -> ()
      }
    }
  }
  n226 = Release Queue(queue=w4, error in (no error)=w2) -> (error out=w5:errorcluster)  [unwired: 1 in, 2 out]
  n227 = Release Queue(queue=w3, error in (no error)=w5) -> ()  [unwired: 1 in, 3 out]
